vi "AB_API Create ProgressBar Events.vi"(8 "error in (no error)":errorcluster) -> (0 "error out":errorcluster, 3 "progressBarEvents":T1)   [LabVIEW 2020]
uses:
  <resource>/Framework/Providers/Common/provcom_ProgressBar_Events.ctl
  <resource>/Framework/Providers/API/mxLvBuildError.ctl
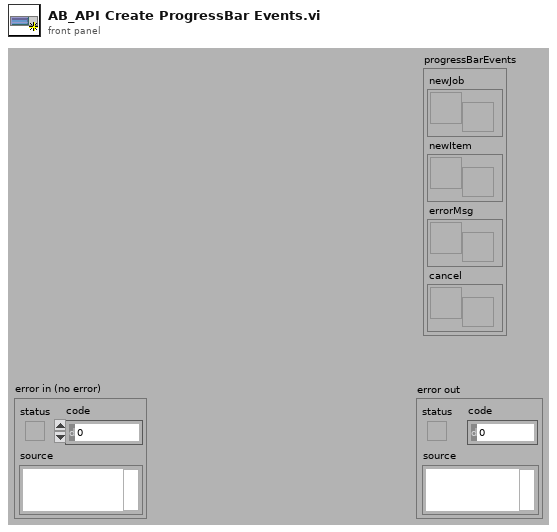
[diagram p1: front panel]
types:
  T1 = typedef "provcom_ProgressBar_Events.ctl" = cluster{"newJob":refnum<user-event>, "newItem":refnum<user-event>, "errorMsg":T2, "cancel":refnum<user-event>}
  T2 = typedef "mxLvBuildError.ctl" = refnum<user-event>
  T3 = typedef "mxLvBuildNewJob.ctl" = refnum<user-event>
  T4 = typedef "mxLvBuildNewItem.ctl" = refnum<user-event>
  T5 = cluster{"NewJob":T3, "NewItem":T4, "Complete":refnum<user-event>}
  T6 = typedef "mxLvBuildCancel.ctl" = refnum<user-event>
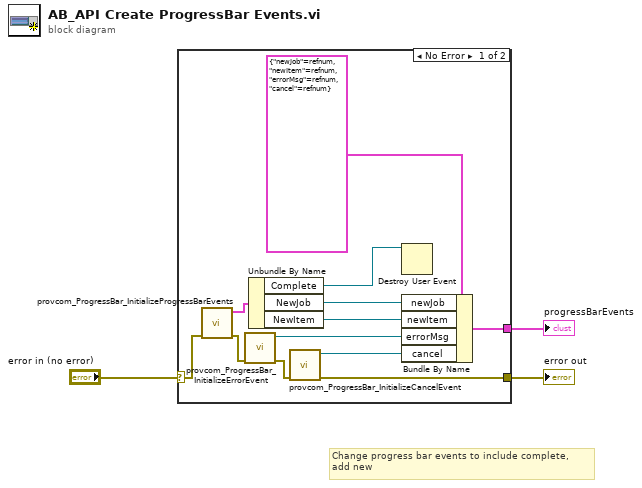
[diagram p0: block diagram]
diagram:
  # "Change progress bar events to include complete, \nadd new"
  n1 = case shown="No Error" "error in (no error)" {
    selector: "error in (no error)" -> [w9 w16]
    tunnel: [w10 _] -> w3
    tunnel: [w5 w16] -> w1
    frame No Error {
      n2 = call <resource>:"provcom_ProgressBar_InitializeProgressBarEvents.vi"("error in (no error)"=w9) -> ("error out"=w8:errorcluster, "ProgressBar events"=w15:T5)  [unwired: 9 in]
      n3 = call <resource>:"provcom_ProgressBar_InitializeErrorEvent.vi"("error in (no error)"=w8) -> ("error out"=w7:errorcluster, "Error event"=w11:T2)  [unwired: 9 in]
      n4 = Unbundle By Name(w15) -> ("Complete"=w4:refnum<user-event>, "NewJob"=w13:T3, "NewItem"=w12:T4)
      n5 = call <resource>:"provcom_ProgressBar_InitializeCancelEvent.vi"("error in (no error)"=w7) -> ("error out"=w5:errorcluster, "Cancel event"=w6:T6)  [unwired: 9 in]
      n6 = Destroy User Event(user event=w4) -> ()  [unwired: 1 in, 1 out]
      n7 = Bundle By Name(cluster=T1 {"newJob"=refnum, "newItem"=refnum, "errorMsg"=refnum, "cancel"=refnum} ("progressBarEvents"), "newJob"=w13, "newItem"=w12, "errorMsg"=w11, "cancel"=w6) -> (w10:T1)
    }
    frame Error {
    }
  }
  "error out" <- w1
  "progressBarEvents" <- w3
